vi "CH1_Comm_TCPIP_NEW.vi"() -> ()   [LabVIEW 2018]
uses:
  RxTx/RxTx.lvclass
panel:
  in  "IP 2":string="200.131.64.49"
  in  "stop":bool
  out "error out 5":errorcluster
  out "error out 4":errorcluster
  out "error out 3":errorcluster
  out "error out 2":errorcluster
  in  "RxTx.lvclass 2":refnum<class "RxTx.lvclass">
  in  "Channel":u16=1
  # "Channel 1 - TCPIP Communication"
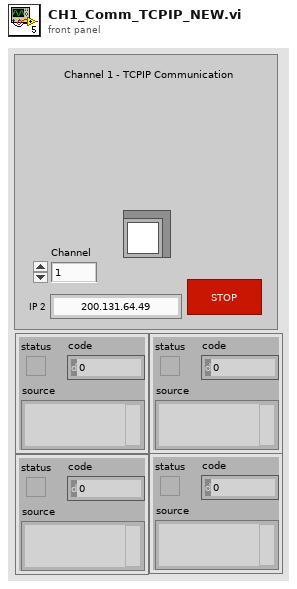
[diagram p1: front panel]
types:
  T1 = enum16{"Standard", "Buffered", "CRLF", "Immediate"}
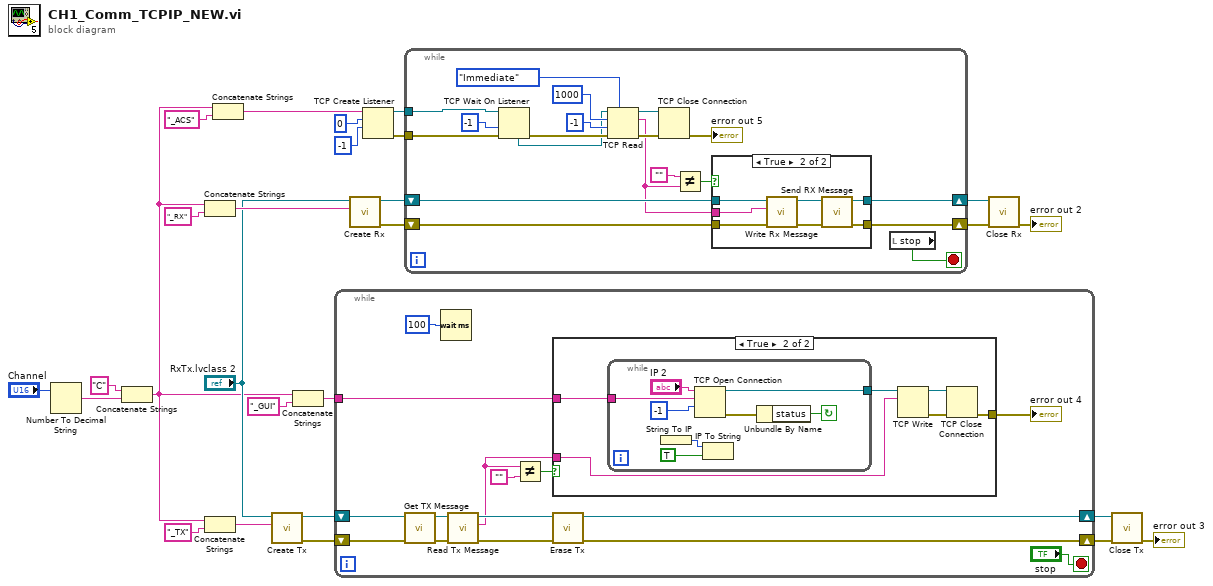
[diagram p0: block diagram]
diagram:
  n1 = Number To Decimal String(number="Channel") -> (decimal integer string=w24:string)  [unwired: 1 in]
  n2 = Concatenate Strings("C", w24) -> (w1:string)
  n3 = Concatenate Strings(w1, "_RX" ("Reader Name")) -> (w27:string)
  n4 = Concatenate Strings(w1, "_TX" ("Reader Name")) -> (w18:string)
  n5 = Concatenate Strings(w1, "_ACS" ("Reader Name")) -> (w6:string)
  n6 = call "Create Tx.vi"("Writer Name"=w18, "RxTx in"="RxTx.lvclass 2") -> ("error out"=w15:errorcluster, "RxTx out"=w16:refnum<class "RxTx.lvclass">)  [unwired: 8 in]
  n7 = Concatenate Strings(w1, "_GUI" ("Reader Name")) -> (w7:string)
  n8 = while {
    shift-right: [w42] -> w14
    shift-left: w16 -> [w35]
    shift-right: [w41] -> w13
    shift-left: w15 -> [w34]
    tunnel: w7 -> [w28]
    stop <- "stop" stop-if-true
    n9 = call "Get TX Message.vi"("error in (no error)"=w34, "RxTx in"=w35) -> ("error out"=w40:errorcluster, "RxTx out"=w36:refnum<class "RxTx.lvclass">)  [unwired: 8 in]
    n10 = Wait (ms)(milliseconds to wait=u32 100) -> ()  [unwired: 1 out]
    n11 = call "Read Tx Message.vi"("error in (no error)"=w40, "RxTx in"=w36) -> ("error out"=w37:errorcluster, "Tx Message"=w29:string, "RxTx out"=w38:refnum<class "RxTx.lvclass">)  [unwired: 7 in]
    n12 = Not Equal?(x=w29, y="") -> (x != y?=w33:bool)
    n13 = case shown="True" w33 {
      tunnel: w29 -> [_ w47]
      tunnel: [_ w43] -> w32
      tunnel: w28 -> [_ w48]
      frame False {
      }
      frame True {
        n14 = while {
          tunnel: w48 -> [w55]
          tunnel: [w52] -> w46
          stop <- w56 continue-if-true
          n15 = String To IP() -> (0:w51:u32)  [unwired: 1 in]
          n16 = TCP Open Connection(address="IP 2", remote port or service name=w55, timeout ms (60000)=-1 ("timeout")) -> (connection ID=w52:refnum<k5>, error out=w54:errorcluster)  [unwired: 2 in]
          n17 = IP To String(1:TRUE ("dot notation? (F)"), 2:w51) -> ()  [unwired: 1 out]
          n18 = Unbundle By Name(w54) -> ("status"=w56:bool)
        }
        n19 = TCP Write(connection ID=w46, data in=w47) -> (connection ID out=w44:refnum<k5>, error out=w45:errorcluster)  [unwired: 2 in, 1 out]
        n20 = TCP Close Connection(connection ID=w44, error in (no error)=w45) -> (error out=w43:errorcluster)  [unwired: 1 in, 1 out]
      }
    }
    "error out 4" <- w32
    n21 = call "Erase Tx.vi"("error in (no error)"=w37, "RxTx in"=w38) -> ("error out"=w41:errorcluster, "RxTx out"=w42:refnum<class "RxTx.lvclass">)  [unwired: 8 in]
  }
  n22 = call "Create Rx.vi"("Reader Name"=w27, "RxTx in"="RxTx.lvclass 2") -> ("error out"=w22:errorcluster, "RxTx out"=w23:refnum<class "RxTx.lvclass">)  [unwired: 8 in]
  n23 = TCP Create Listener(9:-1 ("timeout ms (25000)"), 10:u16 0 ("port"), 11:w6) -> (0:w3:errorcluster, 3:w4:refnum<k5>)  [unwired: 2 in, 1 out]
  n24 = while {
    shift-right: [w70] -> w20
    shift-left: w22 -> [w75]
    shift-right: [w71] -> w21
    shift-left: w23 -> [w74]
    tunnel: w4 -> [w68]
    tunnel: w3 -> [w59]
    stop <- w69 stop-if-true
    n25 = TCP Wait On Listener(8:w59, 9:-1 ("timeout ms (wait forever: -1)"), 11:w68) -> (0:w63:errorcluster, 4:w58:refnum<k5>)  [unwired: 1 in, 3 out]
    n26 = TCP Read(connection ID=w58, bytes to read=1000, error in (no error)=w63, 7:T1."Immediate" ("mode (standard)"), 9:-1 ("timeout ms (25000)")) -> (connection ID out=w61:refnum<k5>, data out=w57:string, error out=w60:errorcluster)
    n27 = TCP Close Connection(connection ID=w61, error in (no error)=w60) -> (error out=→"error out 5":errorcluster)  [unwired: 1 in, 1 out]
    n28 = Not Equal?(x="", y=w57) -> (x != y?=w72:bool)
    n29 = case shown="True" w72 {
      tunnel: w75 -> [w76 w82]
      tunnel: w74 -> [w77 w81]
      tunnel: [w77 w80] -> w71
      tunnel: [w76 w79] -> w70
      tunnel: w57 -> [_ w78]
      frame False {
      }
      frame True {
        n30 = call "Write Rx Message.vi"("error in (no error)"=w82, "Rx Message"=w78, "RxTx in"=w81) -> ("error out"=w83:errorcluster, "RxTx out"=w84:refnum<class "RxTx.lvclass">)  [unwired: 7 in]
        n31 = call "Send RX Message.vi"("error in (no error)"=w83, "RxTx in"=w84) -> ("error out"=w79:errorcluster, "RxTx out"=w80:refnum<class "RxTx.lvclass">)  [unwired: 8 in]
      }
    }
    n32 = local read "stop"() -> (w69:bool)
  }
  n33 = call "Close Rx.vi"("error in (no error)"=w20, "RxTx in"=w21) -> ("error out"=→"error out 2":errorcluster)  [unwired: 8 in, 1 out]
  n34 = call "Close Tx.vi"("error in (no error)"=w13, "RxTx in"=w14) -> ("error out"=→"error out 3":errorcluster)  [unwired: 8 in, 1 out]
